vi "CalcTimeDifference_ms.vi"(7 "ReadOnlyIm":T1={"Qref"={"ValveCTR"=refnum, "Error"=refnum}, "UI_EN"=FALSE, "UserEventREF"={"TimeBasedProducer"={"Reg"=refnum, "Ref"=refnum}, "TimeBasedTempRead"={"Reg"=refnum, "Ref"=refnum}}, "UI_REF"=variant, "Paths"={"Log_Dir"=path "", "TempLog"=path "", "WateringLog"=path "", "Error"=path "", "Settings_Dir"=path "", "CFG.ini"=path "", "Plant_Digital_OP"=path "", "TimeTable"=path "", "Consol_Dir"=path "", "Input"=path "", "Output"=path "", "Timeout"=path "", "TimeoutTable"=path "", "Ch_Stat"=path "", "Temp"=path ""}, "PI_REF"={"IO"=enum."Remote", "Interface"=enum."Serial", "LINX Device Config"={"Interface"=enum."Serial", "COM Port"="COM13", "TCP Configuration"={"IP Address"="", "Port"=0}, "Device Family"=1, "Device ID"=1, "Device Name"="myRIO-1900", "TCP Ref"=refnum, "Channels"={"DI"=[0, 1, 2, 3, 4, 5, 6, 7, 8, 9, 10, 11, 12, 13, 14, 15, 16, 17, 18, 19, 20, 21, 22, 23, 24, 25, 26, 27, 28, 29, 30, 31, 32, 33, 34, 35, 36, 37, 38, 39, 40, 41, 42, 43, 44, 45, 46], "DO"=[0, 1, 2, 3, 4, 5, 6, 7, 8, 9, 10, 11, 12, 13, 14, 15, 16, 17, 18, 19, 20, 21, 22, 23, 24, 25, 26, 27, 28, 29, 30, 31, 32, 33, 34, 35, 36, 37, 38, 39, 40, 41, 42, 43, 44, 45, 46], "AI"=[0, 1, 2, 3, 4, 5, 6, 7, 8, 9, 10, 11], "AO"=[], "PWM"=[3, 5, 6, 9, 10], "QE"=[], "UART"=[0, 1], "I2C 2"=[0], "SPI"=[0], "CAN"=[], "Servo"=[], "AI Ref (V)"=0.0, "AI Resolution (Bits)"=0, "AO Ref (V)"=0.0, "AO Resolution (Bits)"=0}}}, "CFG"={"ProducerEn_PC"=FALSE, "Producer_PC_ms"=0, "ProducerEn_PI"=FALSE, "Producer_PI_ms"=0, "TempLogInterval"=15, "SystemResetTime"=0.0}} {"CFG"."SystemResetTime" format="%<%H:%M:%S>t"}, 8 "Error In":errorcluster, 11 "Read_WriteIN":T9={"Time Table"=[{"Set Time"=0.0, "Control"=enum."Time", "Duration[S]"=3.0, "Liter"=0.0, "Plant Name."="", "Watered"=FALSE, "Su"=FALSE, "Mo"=FALSE, "Tu"=FALSE, "We"=FALSE, "Th"=FALSE, "Fr"=FALSE, "Sa"=FALSE}, {"Set Time"=0.0, "Control"=enum."Time", "Duration[S]"=5.0, "Liter"=0.0, "Plant Name."="", "Watered"=FALSE, "Su"=FALSE, "Mo"=FALSE, "Tu"=FALSE, "We"=FALSE, "Th"=FALSE, "Fr"=FALSE, "Sa"=FALSE}, {"Set Time"=0.0, "Control"=enum."Time", "Duration[S]"=5.0, "Liter"=0.0, "Plant Name."="", "Watered"=FALSE, "Su"=FALSE, "Mo"=FALSE, "Tu"=FALSE, "We"=FALSE, "Th"=FALSE, "Fr"=FALSE, "Sa"=FALSE}], "Plants_Digital_OP"=[], "delta_ms_w_Index"={"delta_ms"=[], "Index"=[], "RunArray"=[]}, "TimeOutInfo"={"Timeout"=0, "ValveCTR"={"State"=enum."Open Valve", "Channel No"=0, "Duration[S]"=0.0}, "Index"=0}, "LoopName"=""} {"TimeOutInfo"."ValveCTR"."Channel No" items=["7"=7, "11"=11, "12"=12, "13"=13, "15"=15, "16"=16, "18"=18, "29"=29, "32"=32, "33"=33, "35"=35, "36"=36, "37"=37, "38"=38, "40"=40]; "delta_ms_w_Index"."RunArray"."Channel No" items=["7"=7, "11"=11, "12"=12, "13"=13, "15"=15, "16"=16, "18"=18, "29"=29, "32"=32, "33"=33, "35"=35, "36"=36, "37"=37, "38"=38, "40"=40]; "Plants_Digital_OP"."Channel No" items=["7"=7, "11"=11, "12"=12, "13"=13, "15"=15, "16"=16, "18"=18, "29"=29, "32"=32, "33"=33, "35"=35, "36"=36, "37"=37, "38"=38, "40"=40]; "Time Table"."Liter" min=0.0; "Time Table"."Set Time" format="%<%H:%M:%S>t"; "Time Table"."Duration[S]" min=0.0}) -> (0 "Error Out":errorcluster, 2 "delta_Sec":i32[](array[numeric]), 3 "Read_WriteOUT":T9={"Time Table"=[{"Set Time"=0.0, "Control"=enum."Time", "Duration[S]"=3.0, "Liter"=0.0, "Plant Name."="", "Watered"=FALSE, "Su"=FALSE, "Mo"=FALSE, "Tu"=FALSE, "We"=FALSE, "Th"=FALSE, "Fr"=FALSE, "Sa"=FALSE}, {"Set Time"=0.0, "Control"=enum."Time", "Duration[S]"=5.0, "Liter"=0.0, "Plant Name."="", "Watered"=FALSE, "Su"=FALSE, "Mo"=FALSE, "Tu"=FALSE, "We"=FALSE, "Th"=FALSE, "Fr"=FALSE, "Sa"=FALSE}, {"Set Time"=0.0, "Control"=enum."Time", "Duration[S]"=5.0, "Liter"=0.0, "Plant Name."="", "Watered"=FALSE, "Su"=FALSE, "Mo"=FALSE, "Tu"=FALSE, "We"=FALSE, "Th"=FALSE, "Fr"=FALSE, "Sa"=FALSE}], "Plants_Digital_OP"=[], "delta_ms_w_Index"={"delta_ms"=[], "Index"=[], "RunArray"=[]}, "TimeOutInfo"={"Timeout"=0, "ValveCTR"={"State"=enum."Open Valve", "Channel No"=0, "Duration[S]"=0.0}, "Index"=0}, "LoopName"=""} {"TimeOutInfo"."ValveCTR"."Channel No" items=["7"=7, "11"=11, "12"=12, "13"=13, "15"=15, "16"=16, "18"=18, "29"=29, "32"=32, "33"=33, "35"=35, "36"=36, "37"=37, "38"=38, "40"=40]; "delta_ms_w_Index"."RunArray"."Channel No" items=["7"=7, "11"=11, "12"=12, "13"=13, "15"=15, "16"=16, "18"=18, "29"=29, "32"=32, "33"=33, "35"=35, "36"=36, "37"=37, "38"=38, "40"=40]; "Plants_Digital_OP"."Channel No" items=["7"=7, "11"=11, "12"=12, "13"=13, "15"=15, "16"=16, "18"=18, "29"=29, "32"=32, "33"=33, "35"=35, "36"=36, "37"=37, "38"=38, "40"=40]; "Time Table"."Liter" min=0.0; "Time Table"."Set Time" format="%<%H:%M:%S>t"; "Time Table"."Duration[S]" min=0.0})   [LabVIEW 2021, in "TimeBasedProd.lvlib"]
uses:
  TimeBasedProd.lvlib
  TypeDef/Read_Write.ctl
  TimeTable/TypeDef/Time_Table.ctl
  TimeTable/TypeDef/Time_Table_CTR.ctl
  Digital_OP/TypeDef/Plant_OP_Map.ctl
  Digital_OP/TypeDef/Plant_OP_Map_CTR.ctl
  ValveCTRL/TypeDef/CHs_List.ctl
  TypeDef/TimeOutInfo.ctl
  ValveCTRL/TypeDef/Queue_Cluster.ctl
  ValveCTRL/TypeDef/States_Enum.ctl
  TypeDef/UpdateTimeOutinfo.ctl
  Main/TypeDef/ReadOnly.ctl
  Main/TypeDef/EventData.ctl
  <vilib>/MakerHub/LINX/Private/Type Defs/LINX Ref.ctl
  <vilib>/MakerHub/LINX/Private/Type Defs/Platform.ctl
  <vilib>/MakerHub/LINX/Private/Type Defs/Interface.ctl
  <vilib>/MakerHub/LINX/Private/Device/Type Defs/LINX Device Config.ctl
  <vilib>/MakerHub/LINX/Private/Device/Type Defs/TCP Config.ctl
  <vilib>/MakerHub/LINX/Private/Device/Type Defs/Channels.ctl
  Main/Init/ReadInitCFG/TypeDef/CFG_Cluster.ctl
  Digital_OP/Plant_Name_to_CH.vi
  ValveCTRL/ValveCTRL.lvlib
  Time/Time.lvlib
  Main/Main.lvlib
  <vilib>/MakerHub/LINX/LMH-LINX.lvlib
  <vilib>/MakerHub/LINX/Private/Device/Device.lvlib
panel:
  out "Local Date Time":string
  # "Watering Days"
  # "Watering Days"
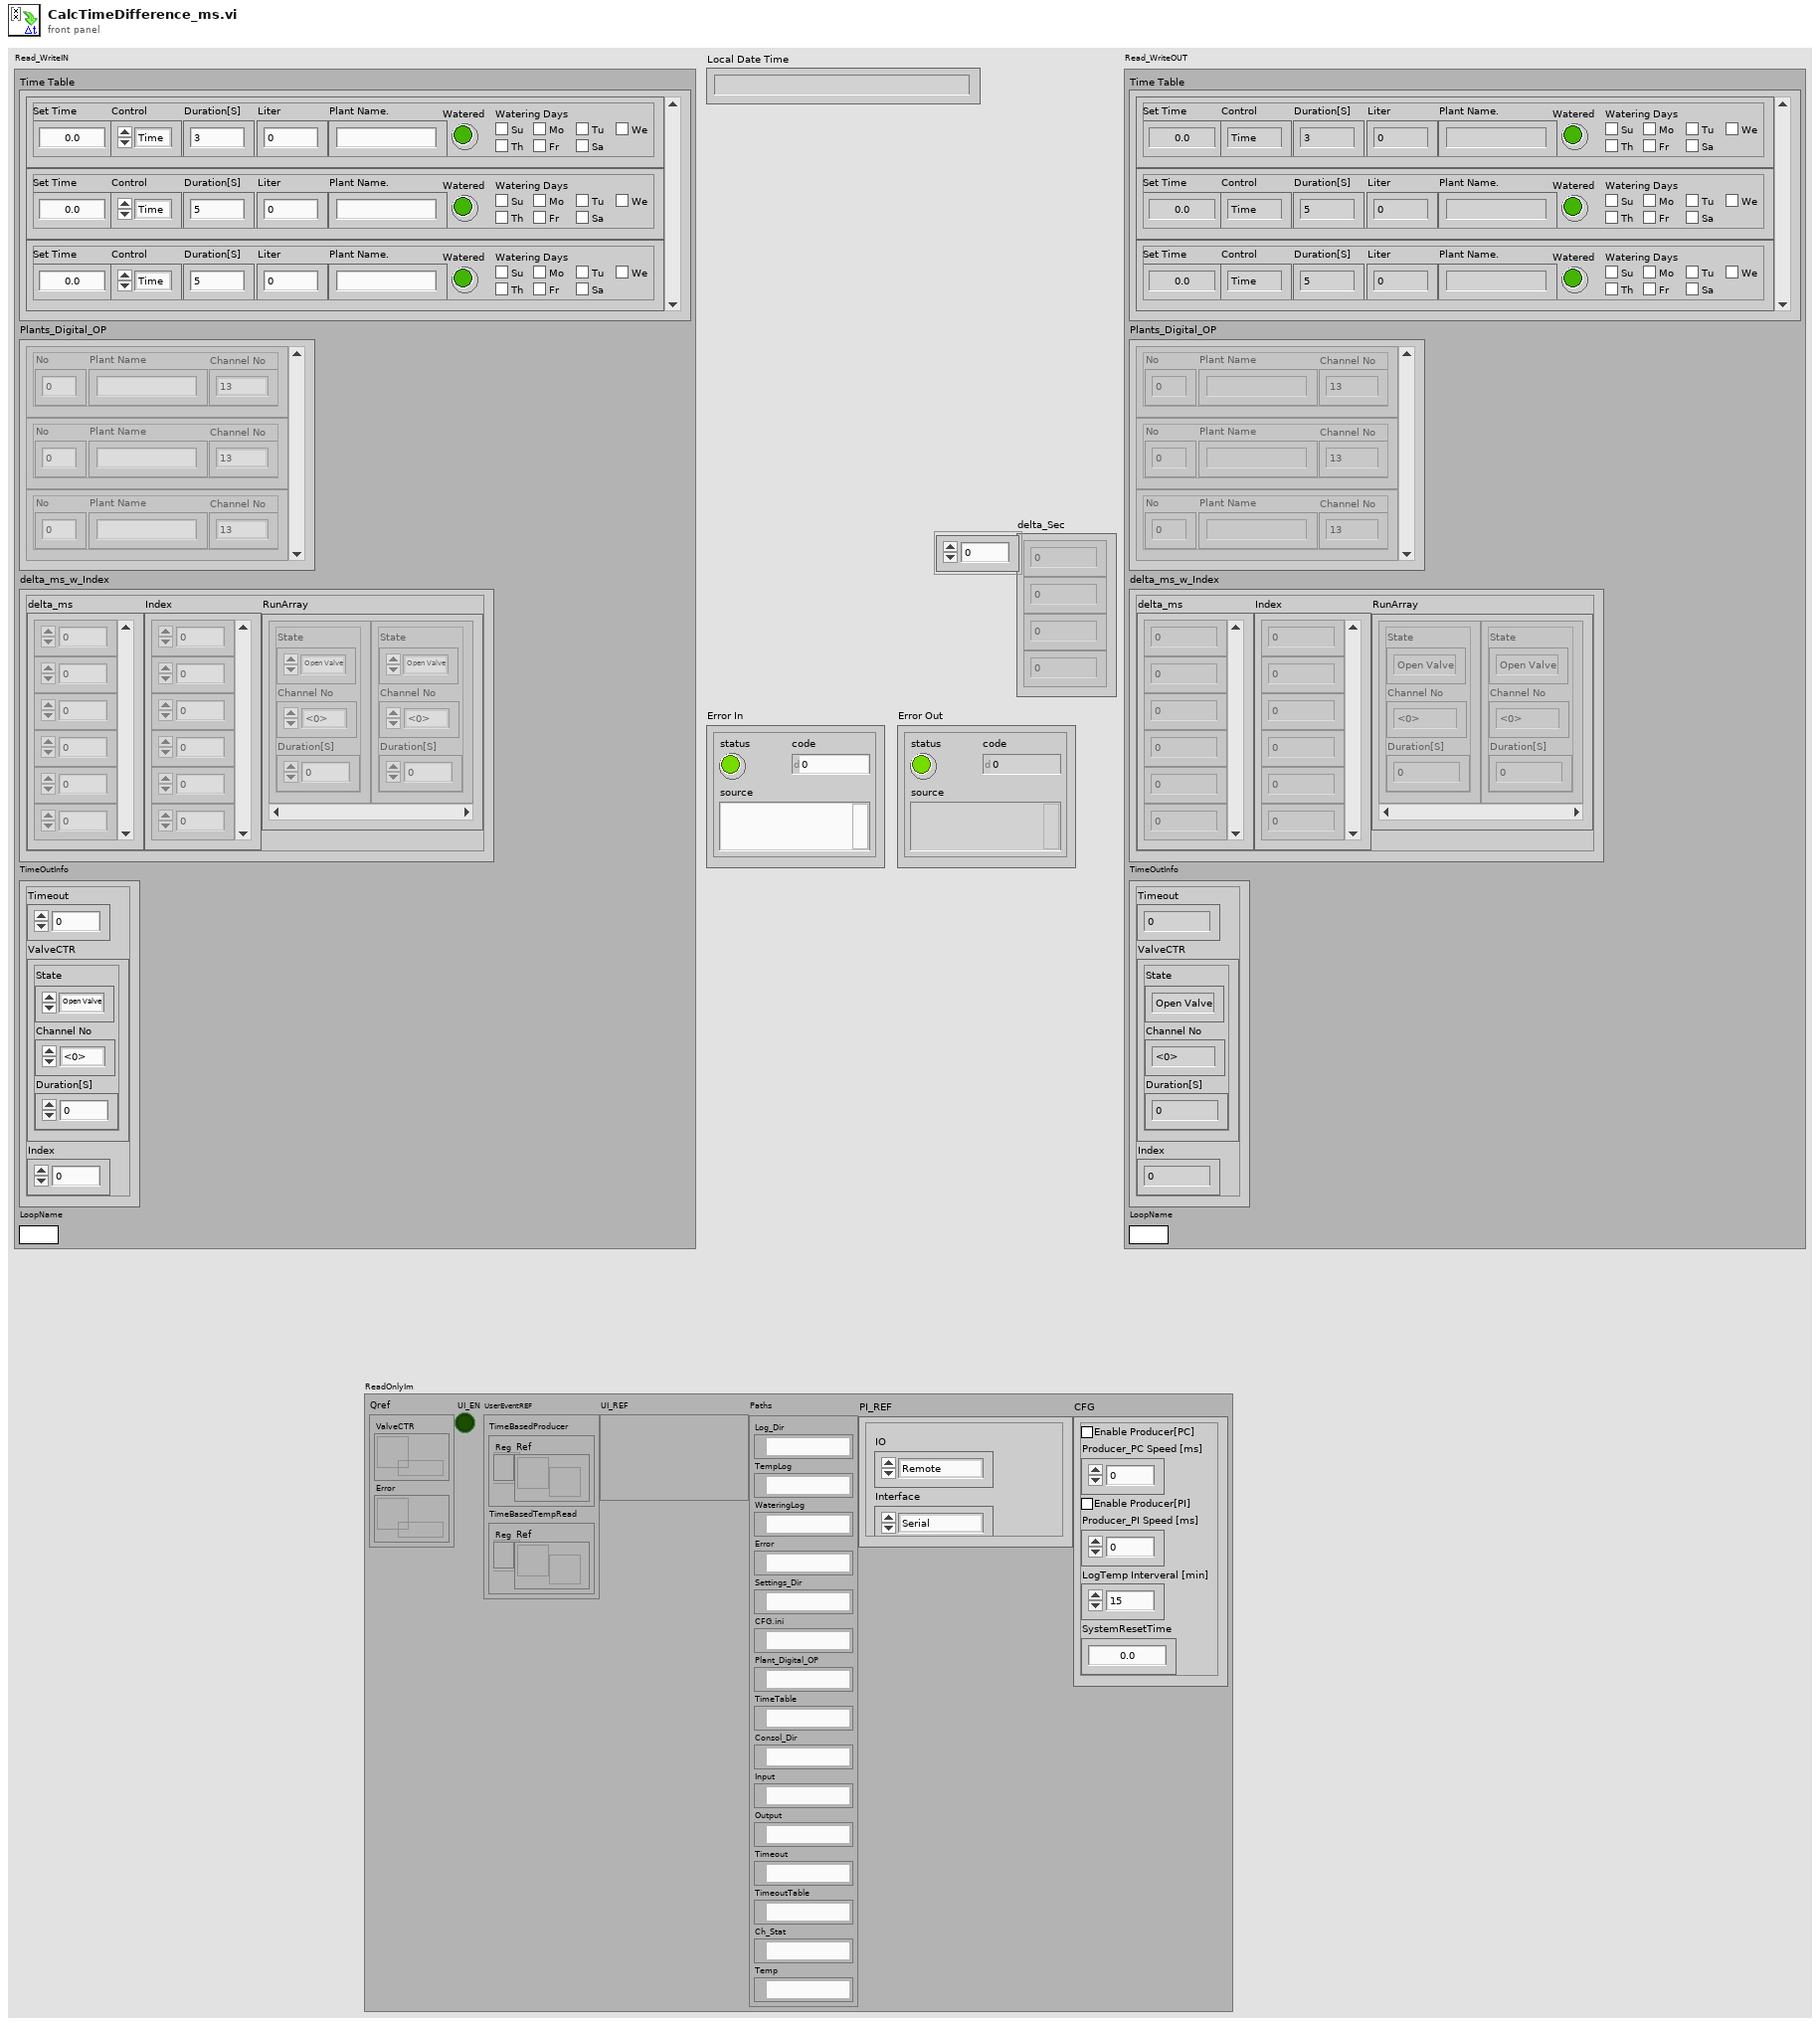
[diagram p1: front panel]
types:
  T1 = typedef "Main.lvlib/ReadOnly.ctl" = cluster{"Qref":cluster{"ValveCTR":refnum<queue>, "Error":refnum<queue>}, "UI_EN":bool, "UserEventREF":cluster{"TimeBasedProducer":cluster{"Reg":refnum<event-registration>, "Ref":refnum<user-event>}, "TimeBasedTempRead":cluster{"Reg":refnum<event-registration>, "Ref":refnum<user-event>}}, "UI_REF":variant, "Paths":cluster{"Log_Dir":path, "TempLog":path, "WateringLog":path, "Error":path, "Settings_Dir":path, "CFG.ini":path, "Plant_Digital_OP":path, "TimeTable":path, "Consol_Dir":path, "Input":path, "Output":path, "Timeout":path, "TimeoutTable":path, "Ch_Stat":path, "Temp":path}, "PI_REF":T2, "CFG":T8}
  T2 = typedef "LMH-LINX.lvlib/LINX Ref.ctl" = cluster{"IO":T3, "Interface":T4, "LINX Device Config":T5}
  T3 = typedef "LMH-LINX.lvlib/Platform.ctl" = enum16{"Remote", "Local"}
  T4 = typedef "LMH-LINX.lvlib/Interface.ctl" = enum16{"Serial", "TCP"}
  T5 = typedef "LMH-LINX.lvlib/Device.lvlib/LINX Device Config.ctl" = cluster{"Interface":T4, "COM Port":refnum<visa-resource-name>, "TCP Configuration":T6, "Device Family":u8, "Device ID":u8, "Device Name":string, "TCP Ref":refnum<k5>, "Channels":T7}
  T6 = typedef "LMH-LINX.lvlib/Device.lvlib/TCP Config.ctl" = cluster{"IP Address":string, "Port":u16}
  T7 = typedef "LMH-LINX.lvlib/Channels.ctl" = cluster{"DI":u8[], "DO":u8[], "AI":u8[], "AO":u8[], "PWM":u8[], "QE":u8[], "UART":u8[], "I2C 2":u8[], "SPI":u8[], "CAN":u8[], "Servo":u8[], "AI Ref (V)":dbl, "AI Resolution (Bits)":u8, "AO Ref (V)":dbl, "AO Resolution (Bits)":u8}
  T8 = typedef "Main.lvlib/CFG_Cluster.ctl" = cluster{"ProducerEn_PC":bool, "Producer_PC_ms":u32, "ProducerEn_PI":bool, "Producer_PI_ms":u32, "TempLogInterval":u32, "SystemResetTime":dbl}
  T9 = typedef "TimeBasedProd.lvlib/Read_Write.ctl" = cluster{"Time Table":T10, "Plants_Digital_OP":T12, "delta_ms_w_Index":T15, "TimeOutInfo":T18, "LoopName":string}
  T10 = typedef "TimeBasedProd.lvlib/Time_Table.ctl" = T11[]
  T11 = typedef "TimeBasedProd.lvlib/Time_Table_CTR.ctl" = cluster{"Set Time":dbl, "Control":enum16{"Time", "Flow"}, "Duration[S]":dbl, "Liter":dbl, "Plant Name.":string, "Watered":bool, "Su":bool, "Mo":bool, "Tu":bool, "We":bool, "Th":bool, "Fr":bool, "Sa":bool}
  T12 = typedef "TimeBasedProd.lvlib/Plant_OP_Map.ctl" = T13[]
  T13 = typedef "TimeBasedProd.lvlib/Plant_OP_Map_CTR.ctl" = cluster{"No":u8, "Plant Name":string, "Channel No":T14}
  T14 = typedef "ValveCTRL.lvlib/CHs_List.ctl" = u8
  T15 = typedef "TimeBasedProd.lvlib/TimeOutInfo.ctl" = cluster{"delta_ms":i32[], "Index":i32[], "RunArray":T16[]}
  T16 = typedef "ValveCTRL.lvlib/Queue_Cluster.ctl" = cluster{"State":T17, "Channel No":T14, "Duration[S]":dbl}
  T17 = typedef "ValveCTRL.lvlib/States_Enum.ctl" = enum16{"Open Pump", "Open Valve", "Wait Valve", "Close Pump", "Close Valve", "Save State", "StopLoop", "ValidCh"}
  T18 = typedef "TimeBasedProd.lvlib/UpdateTimeOutinfo.ctl" = cluster{"Timeout":i32, "ValveCTR":T16, "Index":i32}
  T19 = enum16{"open", "replace", "create", "open or create", "replace or create", "replace or create with confirmation"}
  T20 = typedef "Time.lvlib/TimeCluster.ctl" = cluster{"Year":i32, "Month":i32, "Day":i32, "Hour":i32, "Min":i32, "Second":i32, "Time[s]":i32, "DayOfWeek":i32}
  T21 = typedef "Time.lvlib/Local_DateTime_String.ctl" = cluster{"Local Date Time":string, "Local Date":string, "Local Time":string}
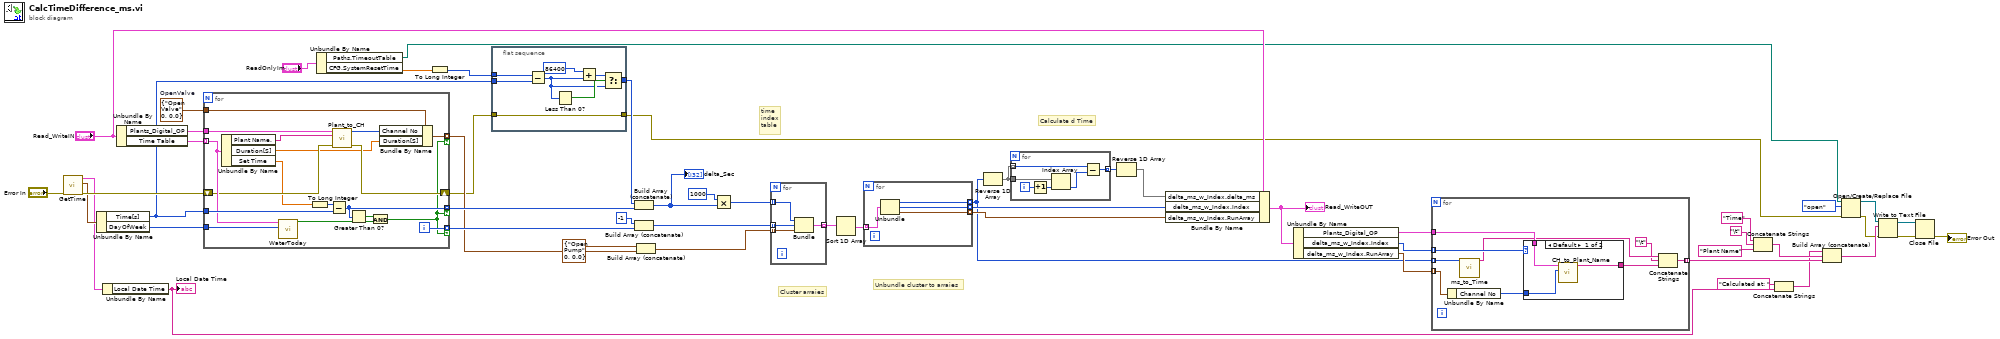
[diagram p0: block diagram]
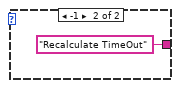
[diagram p2: hidden frame]
diagram:
  w40 = T16 {"State"=enum."Open Valve", "Channel No"=0, "Duration[S]"=0.0}  # OpenValve
  # "time\nindex\ntable"
  # "Calculate d Time"
  # "Unbundle cluster to arraies"
  # "Cluster arraies"
  n1 = call "GetTime.vi"("error in"="Error In") -> ("error out"=w30:errorcluster, "TimeCluster"=w24:T20, "Local Data/Time[String]"=w23:T21)  [unwired: 8 in]
  n2 = Unbundle By Name(w24) -> ("Time[s]"=w28:i32, "DayOfWeek"=w41:i32)
  n3 = Unbundle By Name(w23) -> ("Local Date Time"=w3:string)
  "Local Date Time" <- w3
  n4 = Unbundle By Name("Read_WriteIN") -> ("Plants_Digital_OP"=w36:T12, "Time Table"=w37:T10)
  n5 = for {
    tunnel: w37 -> [w69] mode=indexing
    tunnel: [w71] -> w53 mode=indexing if=w59
    tunnel: w28 -> [w72]
    tunnel: [w70] -> w47 mode=indexing if=w59
    shift-right: [w63] -> w29
    shift-left: w30 -> [w64]
    tunnel: w41 -> [w68]
    tunnel: w40 -> [w62]
    tunnel: [w60] -> w34 mode=indexing if=w59
    tunnel: w36 -> [w58]
    i -> [w70]
    n6 = Unbundle By Name(w69) -> ("Plant Name."=w65:string, "Duration[S]"=w57:dbl, "Set Time"=w56:dbl)
    n7 = call "WaterToday.vi"("Day of week"=w68, "Cluster"=w69) -> ("WaterToday"=w66:bool)  [unwired: 9 in]
    n8 = To Long Integer(number=w56) -> (32bit integer=w55:i32)
    n9 = Subtract(x=w55, y=w72) -> (x-y=w71:i32)
    n10 = call-poly "Plant_to_CH.vi"("Error In"=w64, "Plant Name"=w65, "Plants_Digital_OP"=w58) -> ("Error Out"=w63:errorcluster, "Channel No"=w61:u8)  [unwired: 5 in, 2 out]
    n11 = Greater Than 0?(x=w71) -> (x > 0?=w67:bool)
    n12 = And(x=w67, y=w66) -> (x .and. y?=w59:bool)
    n13 = Bundle By Name(cluster=w62, "Channel No"=w61, "Duration[S]"=w57) -> (w60:T16)
  }
  n14 = Unbundle By Name("ReadOnlyIm") -> ("Paths.TimeoutTable"=w16:path, "CFG.SystemResetTime"=w25:dbl)
  n15 = To Long Integer(number=w25) -> (32bit integer=w27:i32)
  n16 = flat-sequence {
    tunnel: w27 -> [w73]
    tunnel: w28 -> [w80]
    tunnel: [w76] -> w52
    tunnel: w29 -> [w74]
    tunnel: [w74] -> w8
    frame #0 {
      n17 = Subtract(x=w73, y=w80) -> (x-y=w75:i32)
      n18 = Less Than 0?(x=w75) -> (x < 0?=w79:bool)
      n19 = Add(x=86400, y=w75) -> (x+y=w78:i32)
      n20 = Select(t=w78, s=w79, f=w75) -> (s? t:f=w76:i32)
    }
  }
  n21 = Build Array (concatenate)(w52, w53) -> (w45:i32[])
  "delta_Sec" <- w45
  n22 = Build Array (concatenate)(-1, w47) -> (w50:i32[])
  n23 = Build Array (concatenate)(T16 {"State"=enum."Open Pump", "Channel No"=0, "Duration[S]"=0.0}, w34) -> (w33:T16[])
  n24 = Multiply(x=1000, y=w45) -> (x*y=w51:i32[])
  n25 = for {
    tunnel: w51 -> [w84] mode=indexing
    tunnel: w50 -> [w83] mode=indexing
    tunnel: [w82] -> w49 mode=indexing
    tunnel: w33 -> [w81] mode=indexing
    n26 = Bundle(w84, w83, "OpenValve"=w81) -> (w82:cluster{i32, i32, "OpenValve":T16})  [unwired: 1 in]
  }
  n27 = Sort 1D Array(array=w49) -> (sorted array=w48:cluster{i32, i32, "OpenValve":T16}[])
  n28 = for {
    tunnel: [w88] -> w38 mode=indexing
    tunnel: [w87] -> w19 mode=indexing
    tunnel: w48 -> [w86] mode=indexing
    tunnel: [w85] -> w39 mode=indexing
    n29 = Unbundle(w86) -> (w87:i32, w88:i32, "OpenValve"=w85:T16)
  }
  n30 = Reverse 1D Array(array=w19) -> (reversed array=w44:i32[])
  n31 = for {
    tunnel: w44 -> [w90] mode=indexing
    tunnel: w44 -> [w94]
    tunnel: [w91] -> w43 mode=indexing
    i -> [w93]
    n32 = Increment(x=w93) -> (x+1=w92:i32)
    n33 = Index Array(array=w94, index=w92) -> (element=w89:i32)
    n34 = Subtract(x=w90, y=w89) -> (x-y=w91:i32)
  }
  n35 = Reverse 1D Array(array=w43) -> (reversed array=w42:i32[])
  n36 = Bundle By Name(cluster="Read_WriteIN", "delta_ms_w_Index.delta_ms"=w42, "delta_ms_w_Index.Index"=w38, "delta_ms_w_Index.RunArray"=w39) -> (w22:T9)
  "Read_WriteOUT" <- w22
  n37 = Unbundle By Name(w22) -> ("Plants_Digital_OP"=w18:T12, "delta_ms_w_Index.Index"=w21:i32[], "delta_ms_w_Index.RunArray"=w20:T16[])
  n38 = for {
    tunnel: w21 -> [w103] mode=indexing
    tunnel: w19 -> [w102] mode=indexing
    tunnel: w20 -> [w101] mode=indexing
    tunnel: w18 -> [w99]
    tunnel: [w95] -> w17 mode=indexing
    n39 = Unbundle By Name(w101) -> ("Channel No"=w100:T14)
    n40 = call "ms_to_Time.vi"("TimeOut[ms]"=w102) -> ("Time[String]"=w98:string)  [unwired: 10 in]
    n41 = case shown="Default" w103 {
      tunnel: w100 -> [w106 _]
      tunnel: w99 -> [w105 _]
      tunnel: [w104 "Recalculate TimeOut" ("Plant Name")] -> w96
      frame Default {
        n42 = call "CH_to_Plant_Name.vi"("ChannelNo"=w106, "Plants_Digital_OP"=w105) -> ("Plant Name"=w104:string)  [unwired: 8 in, 1 out]
      }
      frame -1 {
      }
    }
    n43 = Concatenate Strings(w98, "\t", w96) -> (w95:string)
  }
  n44 = Concatenate Strings("Time", "\t", "Plant Name") -> (w6:string)
  n45 = Concatenate Strings("Calculated at: " ("string"), w3) -> (w2:string)
  n46 = Build Array (concatenate)(w2, w6, w17) -> (w14:string[])
  n47 = Open/Create/Replace File(file path (use dialog)=w16, error in=w8, operation (0:open)=T19."open") -> (refnum out=w13:refnum<file>, error out=w12:errorcluster)  [unwired: 3 in, 1 out]
  n48 = Write to Text File(file (use dialog)=w13, text=w14, error in=w12) -> (refnum out=w10:refnum<file>, error out=w11:errorcluster)  [unwired: 1 in, 1 out]
  n49 = Close File(refnum=w10, error in=w11) -> (error out=→"Error Out":errorcluster)  [unwired: 1 out]
